vi "SendChatMsg.vi"(8 "error in (no error)":errorcluster, 11 "Server in":refnum<class "Server.lvclass">) -> (0 "error out":errorcluster, 3 "Server out":refnum<class "Server.lvclass">)   [LabVIEW 2021, in "Server.lvlib" / "Server.lvclass"]
uses:
  Server.lvclass
  Server.lvclass/Server.ctl
  Interfaces/Chatter/Chatter Messages/ReceiveChatMsg Msg/ReceiveChatMsg Msg.lvclass/ReceiveChatMsg Msg.ctl
  <vilib>/ActorFramework/Message Enqueuer/Message Enqueuer.lvclass/Message Enqueuer.ctl
  <vilib>/ActorFramework/Message Enqueuer/Enqueue.vi
  Interfaces/Chatter/Chatter Messages/ReceiveChatMsg Msg/ReceiveChatMsg Msg.lvclass
  C:/Program Files/National Instruments/LabVIEW 2021/vi.lib/ActorFramework/Message/Message.lvclass
  <vilib>/ActorFramework/Message Priority Queue/Priority Enqueue.vi
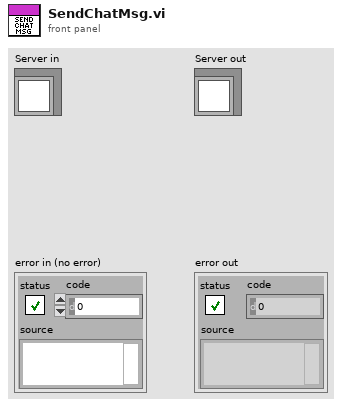
[diagram p1: front panel]
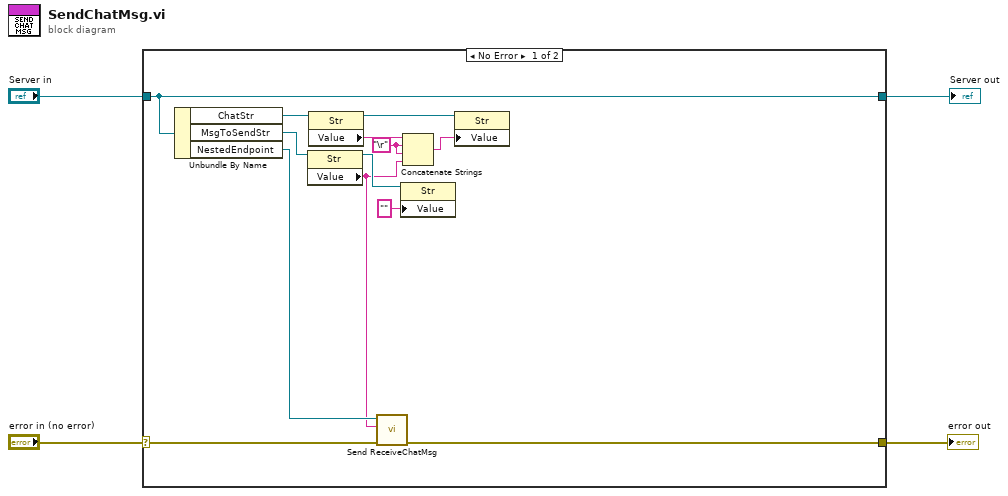
[diagram p0: block diagram]
diagram:
  n1 = case shown="No Error" "error in (no error)" {
    selector: "error in (no error)" -> [w17 w18]
    tunnel: [w7 w18] -> w1
    tunnel: "Server in" -> [w16 w19]
    tunnel: [w16 w19] -> w3
    frame No Error {
      w12 = "\r"
      n2 = Unbundle By Name(w16) -> ("ChatStr"=w15:refnum<vi>, "MsgToSendStr"=w14:refnum<vi>, "NestedEndpoint"=w6:refnum<class "Message Enqueuer.lvclass">)
      n3 = property class="Str"(reference=w14) -> (reference out=w9:refnum<vi>, "Value"=w5:string)  [unwired: 1 in, 1 out]
      n4 = property class="Str"(reference=w15) -> (reference out=w11:refnum<vi>, "Value"=w13:string)  [unwired: 1 in, 1 out]
      n5 = call "Send ReceiveChatMsg.vi"("error in (no error)"=w17, "ChatMsg"=w5, "Message Enqueuer"=w6) -> ("error out"=w7:errorcluster)  [unwired: 7 in, 1 out]
      n6 = property class="Str"(reference=w9, "Value"="") -> ()  [unwired: 1 in, 2 out]
      n7 = Concatenate Strings(w13, w12, w12, w5) -> (w10:string)
      n8 = property class="Str"(reference=w11, "Value"=w10) -> ()  [unwired: 1 in, 2 out]
    }
    frame Error {
    }
  }
  "error out" <- w1
  "Server out" <- w3
